vi "Time.vi"(11 "Output All":string) -> (3 "Time (24h)":string)   [LabVIEW 2015]
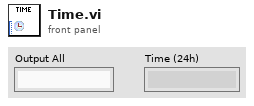
[diagram p1: front panel]
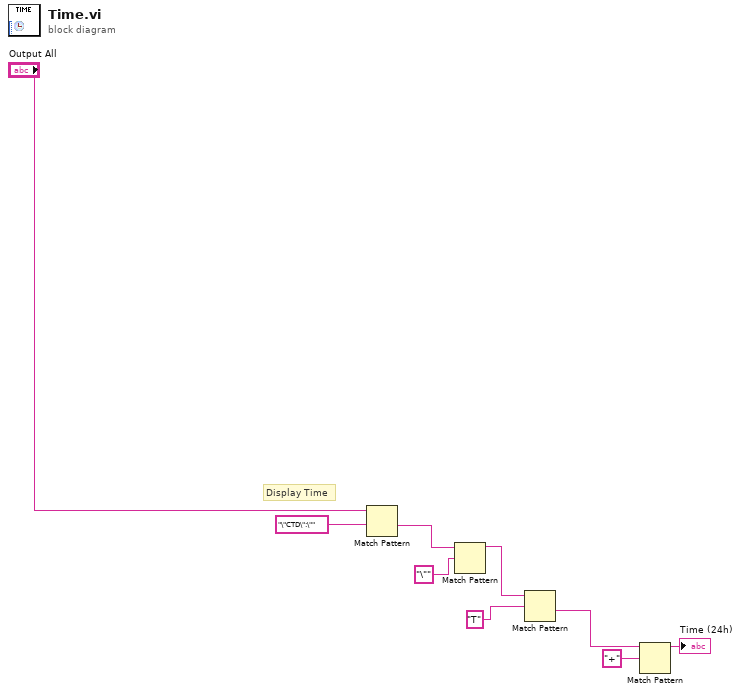
[diagram p0: block diagram]
diagram:
  # "Display Time"
  n1 = Match Pattern(string="Output All", regular expression="\"CTD\":\"") -> (after substring=w8:string)  [unwired: 1 in, 3 out]
  n2 = Match Pattern(string=w8, regular expression="\"") -> (before substring=w5:string)  [unwired: 1 in, 3 out]
  n3 = Match Pattern(string=w5, regular expression="T") -> (after substring=w1:string)  [unwired: 1 in, 3 out]
  n4 = Match Pattern(string=w1, regular expression="+") -> (before substring=→"Time (24h)":string)  [unwired: 1 in, 3 out]
